vi "DaQ_Signal.vi"(8 "Error In":errorcluster, 10 "Signal":waveform(dbl), 11 "Queue In":refnum<queue>) -> (0 "Error Out":errorcluster, 3 "Queue Out":refnum<queue>)   [LabVIEW 2021]
doc: "This subVI is used to enqueue the signal value."
panel:
  # "Input"
  # "Output"
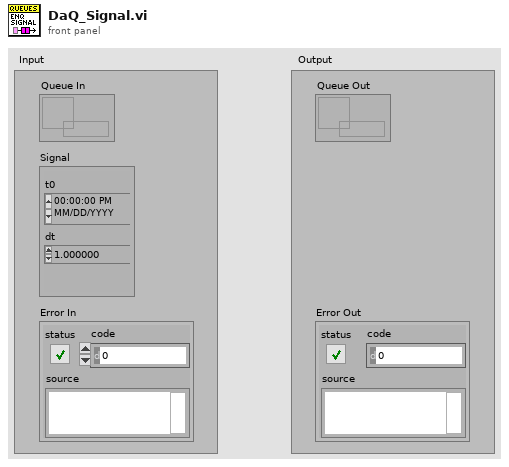
[diagram p1: front panel]
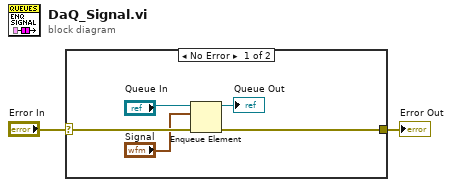
[diagram p0: block diagram]
diagram:
  n1 = case shown="No Error" "Error In" {
    selector: "Error In" -> [w7 w8]
    tunnel: [w3 w8] -> w1
    frame No Error {
      n2 = Enqueue Element(queue="Queue In", element="Signal", error in (no error)=w7) -> (queue out=→"Queue Out":refnum<queue>, error out=w3:errorcluster)  [unwired: 1 in, 1 out]
    }
    frame Error {
    }
  }
  "Error Out" <- w1
